vi "Assert Scalar wired to Scalar Type.vi"   [LabVIEW 2017]
uses:
  f0d9073c-ab1a-44fa-a217-cbc10906d5c2.vi
  88fa0d59-58d3-4d6c-8022-4989553e5c3b.vi
  bb9ddca5-ce9d-4f2b-8cd6-ed48185ca9bb.vi
  76190fae-5e6e-40b7-9495-4e549a90d0b3.vi
  cd9e7d6e-2906-4e4d-9043-47c52e9d418b.vi
  f0d9073c-ab1a-44fa-a217-cbc10906d5c2.vi/0729ff7c-c5ea-47df-910c-98d3e138407c.vi
  88fa0d59-58d3-4d6c-8022-4989553e5c3b.vi/c100a3a4-0ce4-4533-b029-434831e2079b.vi
  bb9ddca5-ce9d-4f2b-8cd6-ed48185ca9bb.vi/313fb904-0ea4-42e4-9466-baffa90e9bca.vi
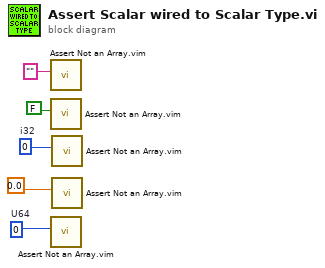
[diagram p0: block diagram]
diagram:
  w1 = u64 0  # U64
  w3 = 0  # i32
  n1 = call "Assert Not an Array.vim"("Input"="") -> ()  [unwired: 10 in, 1 out]
  n2 = call "Assert Not an Array.vim"("Input"=FALSE) -> ()  [unwired: 10 in, 1 out]
  n3 = call "Assert Not an Array.vim"("Input"=w1) -> ()  [unwired: 10 in, 1 out]
  n4 = call "Assert Not an Array.vim"("Input"=w3) -> ()  [unwired: 10 in, 1 out]
  n5 = call "Assert Not an Array.vim"("Input"=0.0) -> ()  [unwired: 10 in, 1 out]
